vi "Register UIMessage Callbacks.vi"(6 "UIMessage IDs":T1[](array[typedef]), 7 "Owner":refnum<class>, 8 "error in (no error)":errorcluster, 9 "User Data":variant, 10 "Callback":T2, 11 "Engine in":refnum<class "Engine.lvclass">) -> (0 "error out":errorcluster, 2 "Callback ID":i32, 3 "Engine out":refnum<class "Engine.lvclass">)   [LabVIEW 2020, in "TSnax.lvlib" / "Engine.lvclass"]
uses:
  Engine.lvclass
  UIMsg Callback VI.ctl
  UIMessage/UIMessage.lvclass
  UIMsg.ctl
  UIMessage Callback.ctl
  Engine.lvclass/Engine.ctl
  <vilib>/Utility/miscctls.llb/LVMapReplaceAction.ctl
  TSnax.lvlib
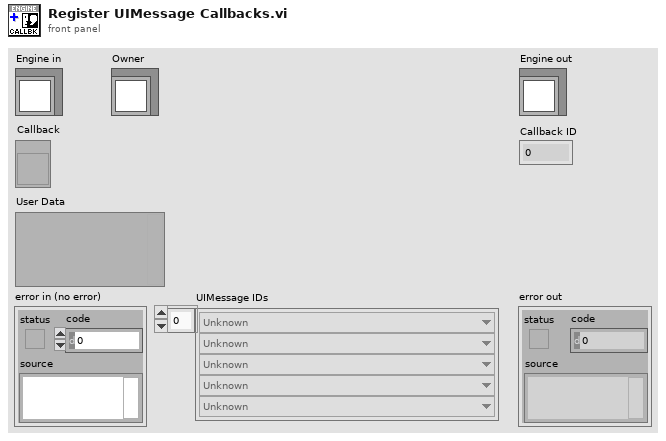
[diagram p1: front panel]
types:
  T1 = typedef "TSnax.lvlib/UIMsg.ctl" = enum16{"Unknown", "BreakOnUserRequest", "BreakOnBreakpoint", "BreakOnRunTimeError", "Trace", "TerminatingExecution", "AbortingExecution", "KillingExecutionThreads", "EndExecution", "ShutDownComplete", "StartExecution", "ProgressPercent", "ProgressText", "StartInteractiveExecution", "EndInteractiveExecution", "TerminatingInteractiveExecution", "TerminationCancelled", "ResumeFromBreak", "StartFileExecution", "EndFileExecution", "ShutDownCancelled", "LocalizationSettingChanged", "OpenWindows", "TileWindows", "CascadeWindows", "ReportChanged", "CloseWindows", "RefreshWindows", "ClientFileChanged", "DisplayReport", "ModelState_Initializing", "ModelState_Waiting", "ModelState_Identified", "ModelState_BeginTesting", "ModelState_TestingComplete", "ModelState_PostProcessingComplete", "ModelState_EnabledStateSet", "ReportLocationChanged", "GotoLocation", "PushUndoItem", "OutputMessages", "TypePaletteFileListChanged", "NonTerminatingThreadsArePreventingTermination", "ModelState_PostProcessing", "ReportCollectionChanged", "RuntimeError"}
  T2 = typedef "TSnax.lvlib/Engine.lvclass/UIMsg Callback VI.ctl" = refnum<vi>
  T3 = typedef "TSnax.lvlib/Engine.lvclass/UIMessage Callback.ctl" = cluster{"VI":T2, "Owner":refnum<class>, "User Data":variant, "IDs":T1[]}
  T4 = typedef "LVMapReplaceAction.ctl" = enum32{"Modify Entry only if found", "Add or Modify Entry", "Delete Entry"}
  T5 = typedef "TSnax.lvlib/Engine.lvclass/UIMessage Callbacks.ctl" = cluster{"Callbacks":T3[], "ID Map":map{T1, i32[]}}
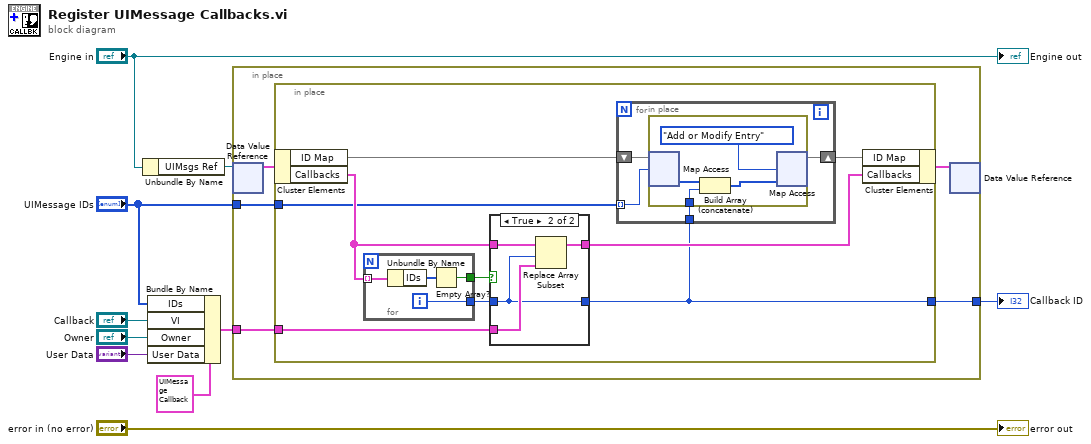
[diagram p0: block diagram]
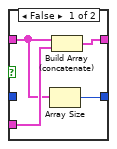
[diagram p2: hidden frame]
diagram:
  n1 = Unbundle By Name("Engine in") -> ("UIMsgs Ref"=w9:refnum<data-value>)
  n2 = Bundle By Name(cluster=T3 {"VI"=refnum, "Owner"=refnum, "User Data"=variant, "IDs"=[]} ("UIMessage Callback"), "IDs"="UIMessage IDs", "VI"="Callback", "Owner"="Owner", "User Data"="User Data") -> (w3:T3)
  n3 = in-place {
    in-place-border: w3 -> [w13]
    in-place-border: "UIMessage IDs" -> [w12]
    in-place-border: [w11] -> w1
    n4 = in-place-dvr #1(w9) -> (w15:T5)  [unwired: 1 out]
    n5 = in-place {
      in-place-border: w13 -> [w21]
      in-place-border: w12 -> [w17]
      in-place-border: [w16] -> w11
      n6 = in-place-cluster #2(w15) -> ("ID Map"=w19:map{T1, i32[]}, "Callbacks"=w22:T3[])
      n7 = for {
        tunnel: w22 -> [w44] mode=indexing
        tunnel: [w42] -> w24
        tunnel: [w41] -> w23
        i -> [w41]
        n8 = Unbundle By Name(w44) -> ("IDs"=w43:T1[])
        n9 = Empty Array?(array=w43) -> (empty?=w42:bool)
      }
      n10 = case shown="True" w24 {
        tunnel: w23 -> [_ w37]
        tunnel: w22 -> [w34 w40]
        tunnel: w21 -> [w36 w38]
        tunnel: [w35 w39] -> w20
        tunnel: [w33 w37] -> w16
        frame False {
          n11 = Array Size(array=w34) -> (size(s)=w33:i32)
          n12 = Build Array (concatenate)(w34, w36) -> (w35:T3[])
        }
        frame True {
          n13 = Replace Array Subset(array=w40, new element=w38, index=w37) -> (w39:T3[])
        }
      }
      n14 = for {
        shift-right: [w25] -> w18
        shift-left: w19 -> [w28]
        tunnel: w17 -> [w27] mode=indexing
        tunnel: w16 -> [w26]
        n15 = in-place {
          in-place-border: w26 -> [w31]
          n16 = in-place-map #3(w28, w27) -> (w32:i32[])  [unwired: 1 in, 1 out]
          n17 = Build Array (concatenate)(w32, w31) -> (w30:i32[])
          n18 = in-place-map #3(w30, LVMapReplaceAction."Add or Modify Entry" ("action")) -> (w25:map{T1, i32[]})  [unwired: 2 out]
        }
      }
      n19 = in-place-cluster #2("ID Map"=w18, "Callbacks"=w20) -> (w14:T5)
    }
    n20 = in-place-dvr #1(w14) -> ()  [unwired: 2 out]
  }
  "Callback ID" <- w1
  "error out" <- "error in (no error)"
  "Engine out" <- "Engine in"
